vi "request.To JSON Tree.vi"(8 "error in (no error)":errorcluster, 11 "Request in":refnum<class "Request.lvclass">) -> (0 "error out":errorcluster, 2 "JSON Value out":variant, 3 "Request out":refnum<class "Request.lvclass">)   [LabVIEW 2020, in "JSON-RPC Lib.lvlib" / "Request.lvclass"]
uses:
  Request.lvclass
  Request.lvclass/Request.ctl
  request.Has ID.vi
  id/id.Read value.vi
  request.has params.vi
  Variant Data Manipulation/Insert Element at Start.vi
  id/id.lvclass
  params/params.lvclass
  Variant Data Manipulation/Variant Data Manipulation.lvlib
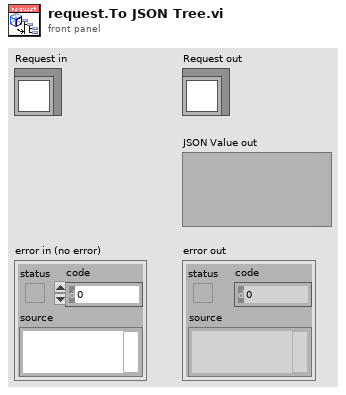
[diagram p1: front panel]
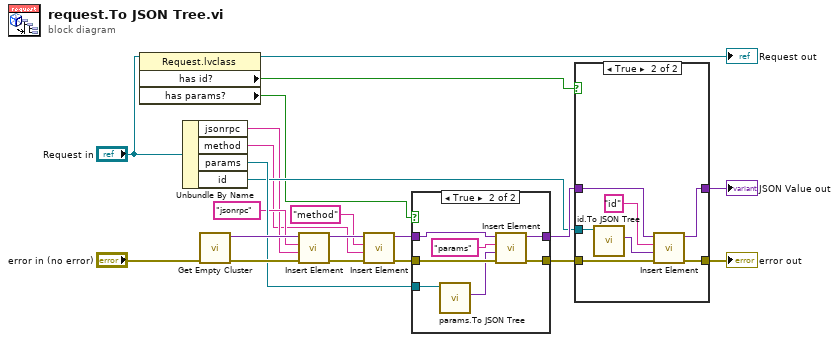
[diagram p0: block diagram]
diagram:
  n1 = property class="Request.lvclass"(reference="Request in") -> (reference out=→"Request out":refnum<class "Request.lvclass">, "has id?"=w10:bool, "has params?"=w6:bool)  [unwired: 1 in, 1 out]
  n2 = Unbundle By Name("Request in") -> ("jsonrpc"=w3:string, "method"=w2:string, "params"=w12:refnum<class "params.lvclass">, "id"=w11:refnum<class "id.lvclass">)
  n3 = call "Get Empty Cluster.vi"("error in (no error)"="error in (no error)") -> ("error out"=w13:errorcluster, "Variant (Cluster) out"=w14:variant)  [unwired: 9 in]
  n4 = call-poly "Insert Element.vi"("error in (no error)"=w13, "element"=w3, "Name"="jsonrpc" ("key"), "Variant (Cluster) in"=w14) -> ("error out"=w19:errorcluster, "Variant (Cluster) out"=w20:variant)  [unwired: 6 in]
  n5 = call-poly "Insert Element.vi"("error in (no error)"=w19, "element"=w2, "Name"="method" ("key"), "Variant (Cluster) in"=w20) -> ("error out"=w17:errorcluster, "Variant (Cluster) out"=w18:variant)  [unwired: 6 in]
  n6 = case shown="True" w6 {
    tunnel: w18 -> [w23 w30]
    tunnel: w17 -> [w22 w29]
    tunnel: [w23 w28] -> w16
    tunnel: [w22 w27] -> w15
    tunnel: w12 -> [_ w26]
    frame False {
    }
    frame True {
      n7 = call "params.To JSON Tree.vi"("params in"=w26) -> ("JSON Value out"=w25:variant)  [unwired: 8 in, 2 out]
      n8 = call-poly "Insert Element.vi"("error in (no error)"=w29, "element"=w25, "Name"="params" ("key"), "Variant (Cluster) in"=w30) -> ("error out"=w27:errorcluster, "Variant (Cluster) out"=w28:variant)  [unwired: 6 in]
    }
  }
  n9 = case shown="True" w10 {
    tunnel: w16 -> [w32 w39]
    tunnel: w15 -> [w31 w38]
    tunnel: w11 -> [_ w37]
    tunnel: [w31 w34] -> w8
    tunnel: [w32 w33] -> w7
    frame False {
    }
    frame True {
      n10 = call "id.To JSON Tree.vi"("id in"=w37) -> ("JSON Value out"=w36:variant)  [unwired: 8 in, 2 out]
      n11 = call-poly "Insert Element.vi"("error in (no error)"=w38, "element"=w36, "Name"="id" ("key"), "Variant (Cluster) in"=w39) -> ("error out"=w34:errorcluster, "Variant (Cluster) out"=w33:variant)  [unwired: 6 in]
    }
  }
  "error out" <- w8
  "JSON Value out" <- w7
